vi "Write PV.vi"(8 "error in (no error)":errorcluster, 10 "PV":refnum<class "PV.lvclass">, 11 "CS++PVUpdate Msg in":refnum<class "CS++PVUpdate Msg.lvclass">) -> (0 "error out":errorcluster, 3 "CS++PVUpdate Msg out":refnum<class "CS++PVUpdate Msg.lvclass">)   [LabVIEW 2012, in "CS++PVMonitor.lvlib" / "CS++PVUpdate Msg.lvclass"]
doc: "Write PV."
uses:
  CS++PVUpdate Msg.lvclass
  Classes/CS++ProcessVariables/ProcessVariable/PV.lvclass
  CS++PVUpdate Msg.lvclass/CS++PVUpdate Msg.ctl
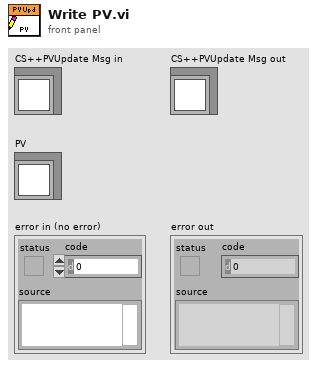
[diagram p1: front panel]
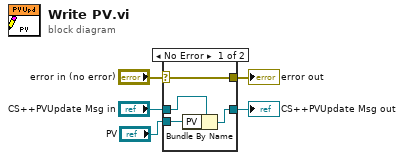
[diagram p0: block diagram]
diagram:
  n1 = case shown="No Error" "error in (no error)" {
    selector: "error in (no error)" -> [w9 w10]
    tunnel: [w9 w10] -> w4
    tunnel: [w7 w11] -> w2
    tunnel: "CS++PVUpdate Msg in" -> [w8 w11]
    tunnel: "PV" -> [w6 _]
    frame No Error {
      n2 = Bundle By Name(cluster=w8, "PV"=w6) -> (w7:refnum<class "CS++PVUpdate Msg.lvclass">)
    }
    frame Error {
    }
  }
  "error out" <- w4
  "CS++PVUpdate Msg out" <- w2
